vi "middleBaseline.vi"   [LabVIEW 2016]
uses:
  <vilib>/Rock Robotics/WPI/ThirdParty/CanMotor/TalonSRX/WPI_CANTalonSRX_APIControlMode.ctl
  <vilib>/Rock Robotics/WPI/ThirdParty/Sensors/navX/_TypeDefs/FRIC_navX_DeviceNumbersTypeDef.ctl
types:
  T1 = typedef "WPI_CANTalonSRX_APIControlMode.ctl" = enum8{"Percent VBus", "Speed", "Position", "Slave", "Unchanged / Invalid", "Voltage Compensation", "Current", "Motion Profile", "Motion Magic"}
  T2 = typedef "WPI_MotorControlDeviceRef.ctl" = cluster{"DeviceStatus":errorcluster, "Type":T3, "PWM":cluster{"PWM Channel":T4, "DeadBand":T5}, "CAN":cluster{"Device Number":u8, "SetOutput VI Ref":variant, "GetOutput VI Ref":variant, "Enable VI Ref":variant, "Disable VI Ref":variant, "Data":variant}, "Invert":bool}
  T3 = typedef "WPI_MotorControlType.ctl" = enum16{"PWM", "CAN"}
  T4 = typedef "FPGA_DIOPWMChannel.ctl" = enum8{"PWM 0", "PWM 1", "PWM 2", "PWM 3", "PWM 4", "PWM 5", "PWM 6", "PWM 7", "PWM 8", "PWM 9", "PWM MXP 0", "PWM MXP 1", "PWM MXP 2", "PWM MXP 3", "PWM MXP 4", "PWM MXP 5", "PWM MXP 6", "PWM MXP 7", "PWM MXP 8", "PWM MXP 9", "Invalid"}
  T5 = typedef "WPI_PWMDeadband.ctl" = cluster{"Name":string, "maxPositivePwm":i32, "minPositivePwm":i32, "centerPwm":i32, "maxNegativePwm":i32, "minNegativePwm":i32, "angularRange":u16}
  T6 = typedef "WPI_CANTalonSRX_GlobalStatus.ctl" = cluster{"Applied Throttle":dbl, "Module Enabled":bool, "CAN Error":errorcluster, "Closed Loop Error":dbl, "Forward Limit Switch Closed":bool, "Reverse Limit Switch Closed":bool, "Sensor Position":dbl, "Sensor Velocity":dbl, "Current":dbl, "Sticky Fault - Over Temp":bool, "Sticky Fault - Under Voltage":bool, "Sticky Fault - Forward Limit":bool, "Sticky Fault - Reverse Limit":bool, "Sticky Fault - Forward Soft Limit":bool, "Sticky Fault - Reverse Soft Limit":bool, "Brake is Enabled":bool, "Encoder Position":dbl, "Encoder Velocity":dbl, "Encoder Index Count":dbl, "Encoder A Pin State":bool, "Encoder B Pin State":bool, "Encoder Index Pin State":bool, "Analog In":dbl, "Analog In Velocity":dbl, "Temperature (C)":dbl, "Battery Voltage":dbl, "Control 5 Is Supported":bool, "Current Profile Slot Select":dbl, "Pos Div 8":bool, "Vel Div 4":bool, "Pulse Width Position":i32, "Pulse Width Velocity":i32, "Pulse Width Rise To Rise (us)":i32, "Pulse Width Rise To Fall (us)":i32, "Mot Prof Active Is Under Run":bool, "Mot Prof Active Has Under Run":bool, "Mot Prof Active Is Last":bool, "Mot Prof Active Velocity Only":bool, "Mot Prof Active Is Valid":bool, "Mot Prof Buffer Is Full":bool, "Mot Prof Active Profile Slot Select":i32, "Mot Prof NextID":i32, "Mot Prof Count":i32, "Mot Prof Active Velocity":dbl, "Mot Prof Active Position":dbl, "Mot Prof Output Enable":i32}
  T7 = typedef "FRIC_navX_DeviceNumbersTypeDef.ctl" = enum16{"Dev0", "Dev1", "Dev2", "Dev3"}
  T8 = cluster{"Yaw":dbl, "Roll":dbl, "Pitch":dbl, "Heading":dbl, "Fused Heading":dbl}
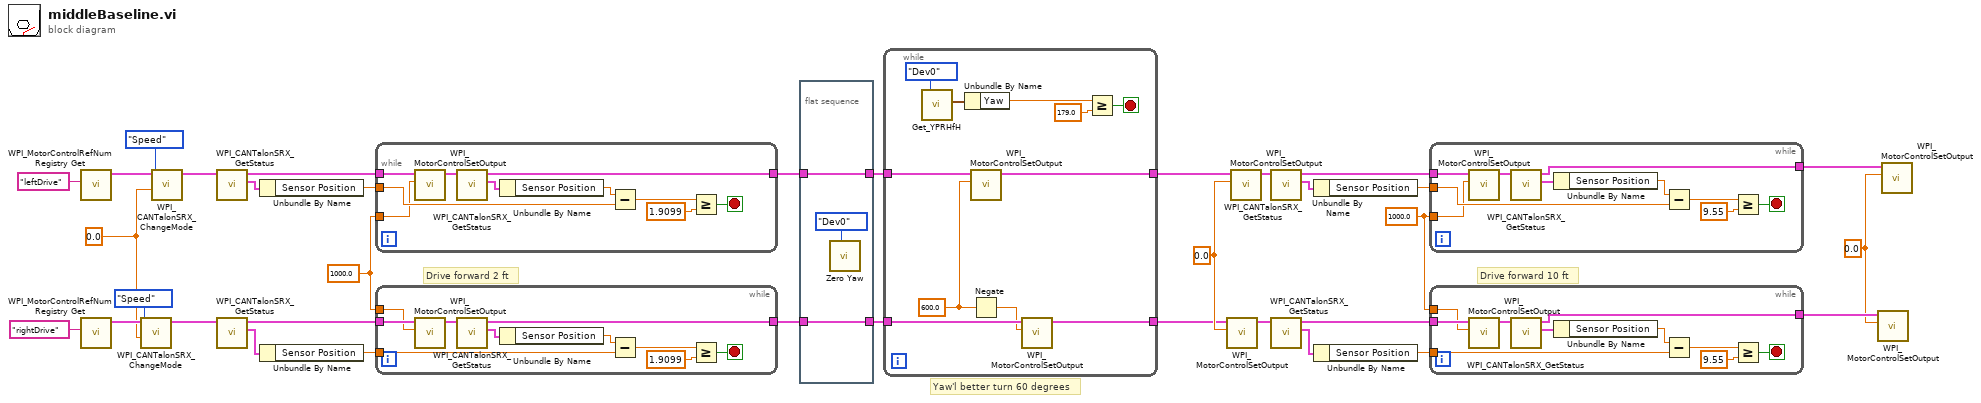
[diagram p0: block diagram]
diagram:
  w5 = 0.0
  w10 = 1000.0
  w17 = 0.0
  w22 = 0.0
  w27 = 1000.0
  # "Drive forward 10 ft"
  # "Drive forward 2 ft"
  # "Yaw'l better turn 60 degrees"
  n1 = call <vilib>:"WPI_MotorControlRefNum Registry Get.vi"("refnum name"="leftDrive") -> ("MotorControlDevRef"=w24:T2)  [unwired: 9 in, 1 out]
  n2 = call <vilib>:"WPI_MotorControlRefNum Registry Get.vi"("refnum name"="rightDrive") -> ("MotorControlDevRef"=w23:T2)  [unwired: 9 in, 1 out]
  n3 = call <vilib>:"WPI_CANTalonSRX_ChangeMode.vi"("Output"=w22, "Control Mode"=WPI_CANTalonSRX_APIControlMode."Speed", "CAN Talon SRX Ref"=w23) -> ("CAN Talon SRX Ref"=w33:T2)  [unwired: 7 in, 1 out]
  n4 = call <vilib>:"WPI_CANTalonSRX_ChangeMode.vi"("Output"=w22, "Control Mode"=WPI_CANTalonSRX_APIControlMode."Speed", "CAN Talon SRX Ref"=w24) -> ("CAN Talon SRX Ref"=w28:T2)  [unwired: 7 in, 1 out]
  n5 = call <vilib>:"WPI_CANTalonSRX_GetStatus.vi"("CAN Talon SRX Ref"=w28) -> ("Talon SRX Status"=w34:T6, "CAN Talon SRX Ref"=w30:T2)  [unwired: 8 in, 1 out]
  n6 = call <vilib>:"WPI_CANTalonSRX_GetStatus.vi"("CAN Talon SRX Ref"=w33) -> ("Talon SRX Status"=w35:T6, "CAN Talon SRX Ref"=w31:T2)  [unwired: 8 in, 1 out]
  n7 = Unbundle By Name(w34) -> ("Sensor Position"=w29:dbl)
  n8 = Unbundle By Name(w35) -> ("Sensor Position"=w32:dbl)
  n9 = while {
    tunnel: w30 -> [w40]
    tunnel: w29 -> [w39]
    tunnel: [w37] -> w7
    tunnel: w27 -> [w36]
    stop <- w38 stop-if-true
    n10 = call <vilib>:"WPI_MotorControlSetOutput.vi"("Output"=w36, "MotorControlDevRef"=w40) -> ("MotorControlDevRef"=w41:T2)  [unwired: 7 in, 2 out]
    n11 = call <vilib>:"WPI_CANTalonSRX_GetStatus.vi"("CAN Talon SRX Ref"=w41) -> ("Talon SRX Status"=w45:T6, "CAN Talon SRX Ref"=w37:T2)  [unwired: 8 in, 1 out]
    n12 = Unbundle By Name(w45) -> ("Sensor Position"=w44:dbl)
    n13 = Subtract(x=w44, y=w39) -> (x-y=w43:dbl)
    n14 = Greater Or Equal?(x=w43, y=1.9099) -> (x >= y?=w38:bool)
  }
  n15 = while {
    tunnel: w32 -> [w53]
    tunnel: w31 -> [w48]
    tunnel: [w47] -> w8
    tunnel: w27 -> [w46]
    stop <- w50 stop-if-true
    n16 = call <vilib>:"WPI_MotorControlSetOutput.vi"("Output"=w46, "MotorControlDevRef"=w48) -> ("MotorControlDevRef"=w49:T2)  [unwired: 7 in, 2 out]
    n17 = call <vilib>:"WPI_CANTalonSRX_GetStatus.vi"("CAN Talon SRX Ref"=w49) -> ("Talon SRX Status"=w55:T6, "CAN Talon SRX Ref"=w47:T2)  [unwired: 8 in, 1 out]
    n18 = Unbundle By Name(w55) -> ("Sensor Position"=w54:dbl)
    n19 = Subtract(x=w54, y=w53) -> (x-y=w52:dbl)
    n20 = Greater Or Equal?(x=w52, y=1.9099) -> (x >= y?=w50:bool)
  }
  n21 = flat-sequence {
    tunnel: [w57] -> w9
    tunnel: w8 -> [w57]
    tunnel: [w56] -> w6
    tunnel: w7 -> [w56]
    frame #0 {
      n22 = call <vilib>:"Zero Yaw.vi"("Device Number"=FRIC_navX_DeviceNumbersTypeDef."Dev0") -> ()  [unwired: 11 in]
    }
  }
  n23 = while {
    tunnel: w6 -> [w65]
    tunnel: w9 -> [w64]
    tunnel: [w61] -> w3
    tunnel: [w60] -> w4
    stop <- w66 stop-if-true
    w63 = 600.0
    n24 = call <vilib>:"Get_YPRHfH.vi"("Device Number"=FRIC_navX_DeviceNumbersTypeDef."Dev0") -> ("YRPHfH"=w69:T8)  [unwired: 10 in]
    n25 = Unbundle By Name(w69) -> ("Yaw"=w68:dbl)
    n26 = call <vilib>:"WPI_MotorControlSetOutput.vi"("Output"=w63, "MotorControlDevRef"=w65) -> ("MotorControlDevRef"=w60:T2)  [unwired: 7 in, 2 out]
    n27 = Negate(x=w63) -> (-x=w62:dbl)
    n28 = call <vilib>:"WPI_MotorControlSetOutput.vi"("Output"=w62, "MotorControlDevRef"=w64) -> ("MotorControlDevRef"=w61:T2)  [unwired: 7 in, 2 out]
    n29 = Greater Or Equal?(x=w68, y=179.0) -> (x >= y?=w66:bool)
  }
  n30 = call <vilib>:"WPI_MotorControlSetOutput.vi"("Output"=w5, "MotorControlDevRef"=w3) -> ("MotorControlDevRef"=w2:T2)  [unwired: 7 in, 2 out]
  n31 = call <vilib>:"WPI_MotorControlSetOutput.vi"("Output"=w5, "MotorControlDevRef"=w4) -> ("MotorControlDevRef"=w1:T2)  [unwired: 7 in, 2 out]
  n32 = call <vilib>:"WPI_CANTalonSRX_GetStatus.vi"("CAN Talon SRX Ref"=w1) -> ("Talon SRX Status"=w15:T6, "CAN Talon SRX Ref"=w12:T2)  [unwired: 8 in, 1 out]
  n33 = call <vilib>:"WPI_CANTalonSRX_GetStatus.vi"("CAN Talon SRX Ref"=w2) -> ("Talon SRX Status"=w16:T6, "CAN Talon SRX Ref"=w13:T2)  [unwired: 8 in, 1 out]
  n34 = Unbundle By Name(w15) -> ("Sensor Position"=w11:dbl)
  n35 = Unbundle By Name(w16) -> ("Sensor Position"=w14:dbl)
  n36 = while {
    tunnel: w12 -> [w74]
    tunnel: w11 -> [w73]
    tunnel: [w71] -> w19
    tunnel: w10 -> [w70]
    stop <- w72 stop-if-true
    n37 = call <vilib>:"WPI_MotorControlSetOutput.vi"("Output"=w70, "MotorControlDevRef"=w74) -> ("MotorControlDevRef"=w75:T2)  [unwired: 7 in, 2 out]
    n38 = call <vilib>:"WPI_CANTalonSRX_GetStatus.vi"("CAN Talon SRX Ref"=w75) -> ("Talon SRX Status"=w79:T6, "CAN Talon SRX Ref"=w71:T2)  [unwired: 8 in, 1 out]
    n39 = Unbundle By Name(w79) -> ("Sensor Position"=w78:dbl)
    n40 = Subtract(x=w78, y=w73) -> (x-y=w77:dbl)
    n41 = Greater Or Equal?(x=w77, y=9.55) -> (x >= y?=w72:bool)
  }
  n42 = while {
    tunnel: w14 -> [w87]
    tunnel: w13 -> [w82]
    tunnel: [w81] -> w18
    tunnel: w10 -> [w80]
    stop <- w84 stop-if-true
    n43 = call <vilib>:"WPI_MotorControlSetOutput.vi"("Output"=w80, "MotorControlDevRef"=w82) -> ("MotorControlDevRef"=w83:T2)  [unwired: 7 in, 2 out]
    n44 = call <vilib>:"WPI_CANTalonSRX_GetStatus.vi"("CAN Talon SRX Ref"=w83) -> ("Talon SRX Status"=w89:T6, "CAN Talon SRX Ref"=w81:T2)  [unwired: 8 in, 1 out]
    n45 = Unbundle By Name(w89) -> ("Sensor Position"=w88:dbl)
    n46 = Subtract(x=w88, y=w87) -> (x-y=w86:dbl)
    n47 = Greater Or Equal?(x=w86, y=9.55) -> (x >= y?=w84:bool)
  }
  n48 = call <vilib>:"WPI_MotorControlSetOutput.vi"("Output"=w17, "MotorControlDevRef"=w18) -> ()  [unwired: 7 in, 3 out]
  n49 = call <vilib>:"WPI_MotorControlSetOutput.vi"("Output"=w17, "MotorControlDevRef"=w19) -> ()  [unwired: 7 in, 3 out]
